vi "ExtractParam.vi"(10 "String":string, 11 "Array":T2(array[cluster])) -> (0 "success?":bool, 1 "1st pt":dbl, 2 "1st Col":dbl[](array[numeric]), 3 "Data":dbl[][](array[numeric]), 4 "complex":bool)   [LabVIEW 2022 SP3]
uses:
  miDataType.ctl
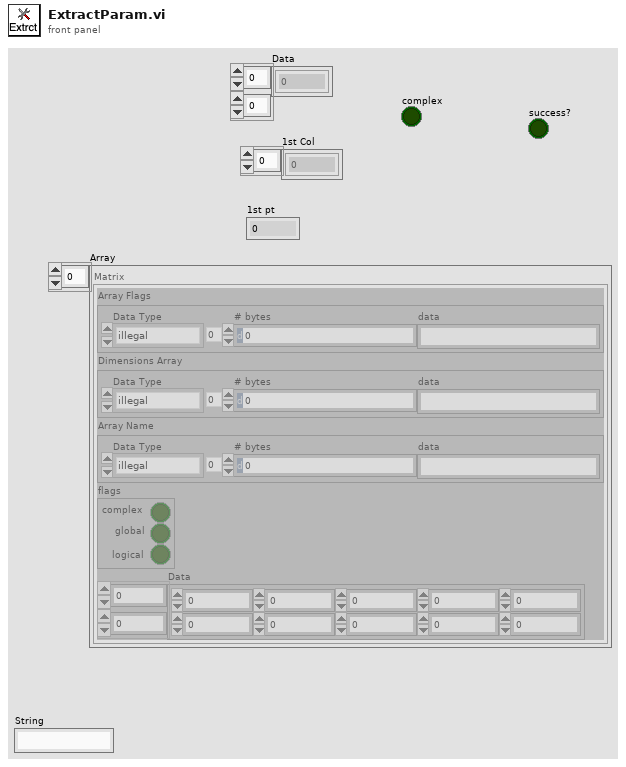
[diagram p1: front panel]
types:
  T1 = typedef "miDataType.ctl" = enum16{"illegal", "miINT8", "miUINT8", "miINT16", "miUINT16", "miINT32", "miUINT32", "miSINGLE", "--", "miDOUBLE", "---", "----", "miINT64", "miUINT64", "miMATRIX", "miCOMPRESSED", "miUTF8", "miUTF16", "miUTF32", "udefined"}
  T2 = cluster{"Array Flags":cluster{"Data Type":T1, "# bytes":u32, "data":string}, "Dimensions Array":cluster{"Data Type":T1, "# bytes":u32, "data":string}, "Array Name":cluster{"Data Type":T1, "# bytes":u32, "data":string}, "flags":cluster{"complex":bool, "global":bool, "logical":bool}, "Data":dbl[][]}[]
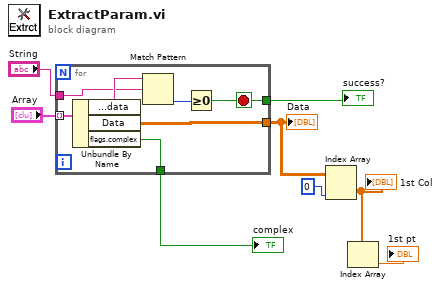
[diagram p0: block diagram]
diagram:
  n1 = for {
    tunnel: "Array" -> [w14] mode=indexing
    tunnel: "String" -> [w11]
    tunnel: [w15] -> w5
    tunnel: [w13] -> w2
    tunnel: [w9] -> w1
    stop <- w9 stop-if-true
    n2 = Unbundle By Name(w14) -> ("Array Name.data"=w12:string, "Data"=w15:dbl[][], "flags.complex"=w13:bool)
    n3 = Match Pattern(string=w12, regular expression=w11) -> (offset past match=w10:i32)  [unwired: 1 in, 3 out]
    n4 = Greater Or Equal To 0?(x=w10) -> (x >= 0?=w9:bool)
  }
  "Data" <- w5
  "complex" <- w2
  "success?" <- w1
  n5 = Index Array(array=w5, index (col)=0 ("index (row)")) -> (element=w4:dbl[])  [unwired: 1 in]
  "1st Col" <- w4
  n6 = Index Array(array=w4) -> (element=→"1st pt":dbl)  [unwired: 1 in]
